vi "Stitching-Setup column selector ring.vi"(11 "Ring in":refnum<vi>) -> (0 "error out":errorcluster)   [LabVIEW 2013]
uses:
  Coordinates list window/Globals/Coord window-Globals.vi
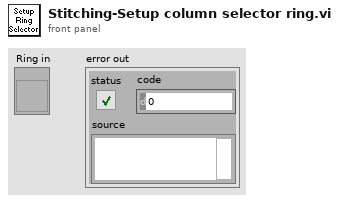
[diagram p1: front panel]
types:
  T1 = typedef "Coordinate list window refs.ctl" = cluster{"Window Name (i.e. Key)":string, "menu reference":refnum<k9>, "VI's reference":refnum<vi>, "Pane 1":refnum<vi>, "Pane 2":refnum<vi>, "Coord Listbox":refnum<vi>, "File name":refnum<vi>, "Picture Map":refnum<vi>, "Stage XYZ Position ind.":refnum<vi>}
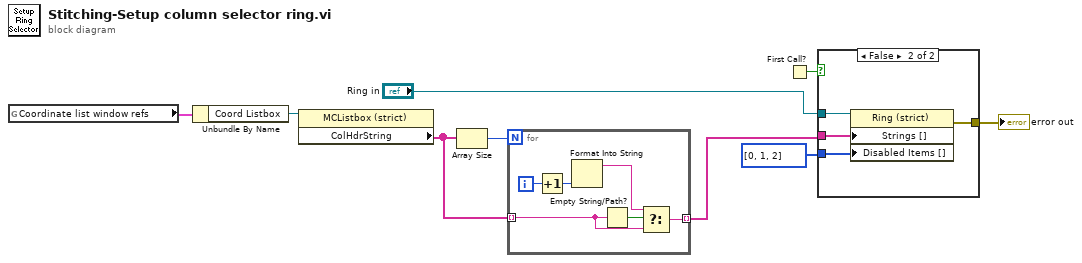
[diagram p0: block diagram]
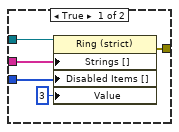
[diagram p2: hidden frame]
diagram:
  n1 = global read "Coord window-Globals.vi" "Coordinate list window refs"() -> (w5:T1)
  n2 = Unbundle By Name(w5) -> ("Coord Listbox"=w6:refnum<vi>)
  n3 = property class="MCListbox (strict)"(reference=w6) -> ("ColHdrString"=w2:string[])  [unwired: 1 in, 2 out]
  n4 = Array Size(array=w2) -> (size(s)=w3:i32)
  n5 = for {
    N: w3 -> [_]
    tunnel: [w10] -> w1 mode=indexing
    tunnel: w2 -> [w12] mode=indexing
    i -> [w15]
    n6 = Increment(x=w15) -> (x+1=w14:i32)
    n7 = Format Into String(w14) -> (resulting string=w11:string)  [unwired: 3 in, 1 out]
    n8 = Empty String/Path?(string/path=w12) -> (empty?=w13:bool)
    n9 = Select(t=w11, s=w13, f=w12) -> (s? t:f=w10:string)
  }
  n10 = First Call?() -> (First Call?: T/F=w9:bool)
  n11 = case shown="False" w9 {
    tunnel: w1 -> [w20 w24]
    tunnel: i32[] [0, 1, 2] ("Disabled Items []") -> [w19 w23]
    tunnel: [w18 w22] -> w8
    tunnel: "Ring in" -> [w16 w21]
    frame True {
      n12 = property on="Property Node" class="Ring (strict)"(reference=w16, "Strings []"=w20, "Disabled Items []"=w19, "Value"=3) -> (error out=w18:errorcluster)  [unwired: 1 in, 1 out]
    }
    frame False {
      n13 = property on="Property Node" class="Ring (strict)"(reference=w21, "Strings []"=w24, "Disabled Items []"=w23) -> (error out=w22:errorcluster)  [unwired: 1 in, 1 out]
    }
  }
  "error out" <- w8
